vi "Write tcp timeouts.vi"(8 "error in (no error)":errorcluster, 9 "write timeout":i32=10000, 10 "read timeout":i32=10000, 11 "Master CR in":refnum<class "Master CR.lvclass">) -> (0 "error out":errorcluster, 3 "Master CR out":refnum<class "Master CR.lvclass">)   [LabVIEW 2021, in "Master CR.lvclass"]
uses:
  Master CR.lvclass
  Master CR.lvclass/Master CR.ctl
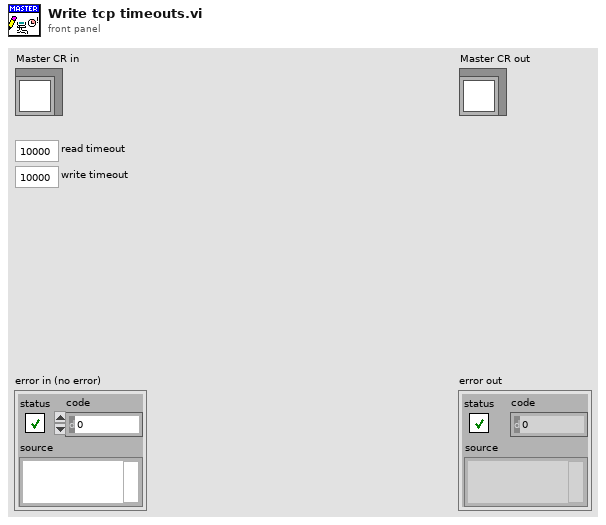
[diagram p1: front panel]
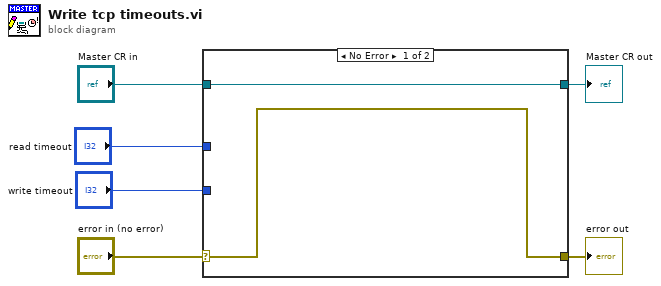
[diagram p0: block diagram]
diagram:
  n1 = case shown="No Error" "error in (no error)" {
    selector: "error in (no error)" -> [w7 w9]
    tunnel: [w7 w9] -> w5
    tunnel: [w8 w10] -> w3
    tunnel: "Master CR in" -> [w8 w10]
    tunnel: "read timeout" -> [_ _]
    tunnel: "write timeout" -> [_ _]
    frame No Error {
    }
    frame Error {
    }
  }
  "error out" <- w5
  "Master CR out" <- w3
